vi "Process.vi"(8 "error in":errorcluster, 11 "UI_Generator_Config":refnum<class "UI_Generator_Config.lvclass">) -> (0 "error out":errorcluster, 3 "UI_Generator_Config out":refnum<class "UI_Generator_Config.lvclass">)   [LabVIEW 2016, in "UI_Generator_Config.lvclass"]
doc: "---------------------------------------------------------------\nJKI State Machine Objects™\nhttp://jki.net/state-machine-objects/\nCopyright (C) 2005-2015, JKI <info@jki.net>\nALL RIGHTS RESERVED"
uses:
  UI_Generator_Config.lvclass
  C:/Program Files (x86)/National Instruments/LabVIEW 2016/vi.lib/JKI/JKI SMO/SMO/SMO.lvclass
  Typedefs/AO-cluster.ctl
  Typedefs/AO_Amp-array.ctl
  Typedefs/AO_DC-array.ctl
  Typedefs/AO_f-array.ctl
  Typedefs/AO_phi-array.ctl
  Typedefs/Function-array.ctl
  Typedefs/Function-enum.ctl
  <vilib>/JKI/JKI SMO/SMO/Typedefs/Parent Call--Enum.ctl
  Generator/Typedefs/PrivateEvents--Generator.configGenerator.ctl
  UI_Generator_Config.lvclass/UI_Generator_Config.ctl
  <vilib>/JKI/JKI SMO/SMO/SMO.lvclass
  Generator/Generator.lvclass
panel:
  in  "Channels: AO":T1={"AO amp (V)"=[0.01, 0.0, 0.0, 0.0, 0.0, 0.0, 0.0, 0.0], "AO DC (V)"=[0.0, 0.0, 0.0, 0.0, 0.0, 0.0, 0.0, 0.0], "AO f (Hz)"=[13.1, 13.0, 13.0, 13.0, 13.0, 13.0, 13.0, 13.0], "AO phi (deg)"=[0.0, 0.0, 0.0, 0.0, 0.0, 0.0, 0.0, 0.0], "function"=[enum."Sine Wave", enum."Sine Wave", enum."Sine Wave", enum."Sine Wave", enum."Sine Wave", enum."Sine Wave", enum."Sine Wave", enum."Sine Wave"]} {"AO f (Hz)" min=0.001 max=10000.0; "AO DC (V)" format="%#_6p"; "AO amp (V)" format="%#_6p"}
  in  "Close Window":bool
  # "For instructions on how to use the JKI State Machine Objects, examples and video tutorials, visit:\nhttp://jki.net/state-machine-objects/\n\nJKI State Machine Objects™\nhttp://jki.net/state-machine-objects/\nCopyright (C) 2005-2015, JKI <info@jki.net>\nALL RIGHTS RESERVED"
  # "I think this UI should update Generator live"
  # "configGenerator"
  # "This VI should initialize by asking Generator\nwhat the current settings are...and populating\nthis controls."
  # "0"
  # "1"
  # "2"
  # "3"
  # "4"
  # "5"
  # "6"
  # "7"
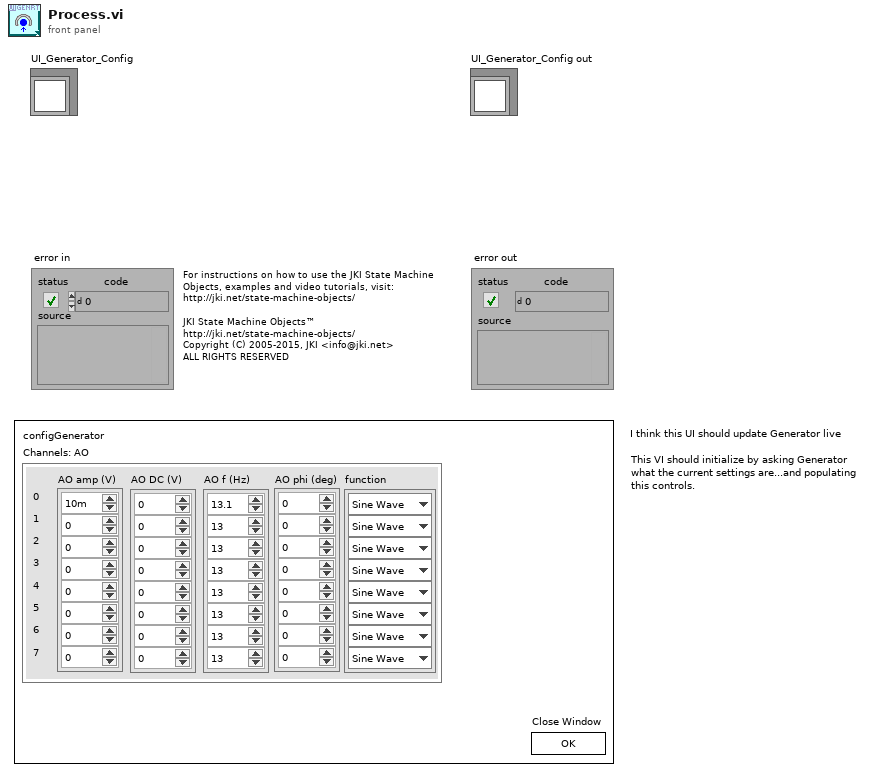
[diagram p1: front panel]
types:
  T1 = typedef "UI_Generator_Config.lvclass/AO-cluster.ctl" = cluster{"AO amp (V)":T2, "AO DC (V)":T3, "AO f (Hz)":T4, "AO phi (deg)":T5, "function":T6}
  T2 = typedef "UI_Generator_Config.lvclass/AO_Amp-array.ctl" = dbl[]
  T3 = typedef "UI_Generator_Config.lvclass/AO_DC-array.ctl" = dbl[]
  T4 = typedef "UI_Generator_Config.lvclass/AO_f-array.ctl" = dbl[]
  T5 = typedef "UI_Generator_Config.lvclass/AO_phi-array.ctl" = dbl[]
  T6 = typedef "UI_Generator_Config.lvclass/Function-array.ctl" = T7[]
  T7 = typedef "UI_Generator_Config.lvclass/Function-enum.ctl" = enum16{"Sine Wave", "Triangle Wave", "Square Wave", "Sawtooth Wave"}
  T8 = cluster{"A (V)":dbl, "DC (V)":dbl, "f (Hz)":dbl, "phi (deg)":dbl, "signal type":enum16{"Sine Wave", "Triangle Wave", "Square Wave", "Sawtooth Wave"}}
  T9 = typedef "SMO.lvclass/Parent Call--Enum.ctl" = enum16{"Allows parent to run", "Does not request parent to run"}
  T10 = enum32{"invalid app kind", "Development System", "Run Time System", "Student Edition", "Embedded LabVIEW", "Evaluation", "Custom"}
  T11 = enum32{"Invalid", "Standard", "Closed", "Hidden", "Minimized", "Maximized"}
  T12 = enum32{"Bad", "Idle", "Run top level", "Running"}
  T13 = typedef "Generator.lvclass/PrivateEvents--Generator.configGenerator.ctl" = cluster{"A (V)":dbl, "DC (V)":dbl, "f (Hz)":dbl, "phi (deg)":dbl, "signal type":enum16{"Sine Wave", "Triangle Wave", "Square Wave", "Sawtooth Wave"}}[]
  T14 = cluster{"Core":cluster{"Current VI Reference":refnum<vi>, "Close Panel on Exit?":bool, "error":errorcluster}, "Self Reference":refnum<class "UI_Generator_Config.lvclass">, "Your string data":string, "configGenerator":T13}
  T15 = cluster{"Current VI Reference":refnum<vi>, "Close Panel on Exit?":bool, "error":errorcluster}
  T16 = typedef "SMO.lvclass/Protected Events.ctl" = cluster{"StopProcesses":refnum<user-event>, "AbortProcesses":refnum<user-event>, "Config Changed":refnum<user-event>, "Dependency":refnum<user-event>}
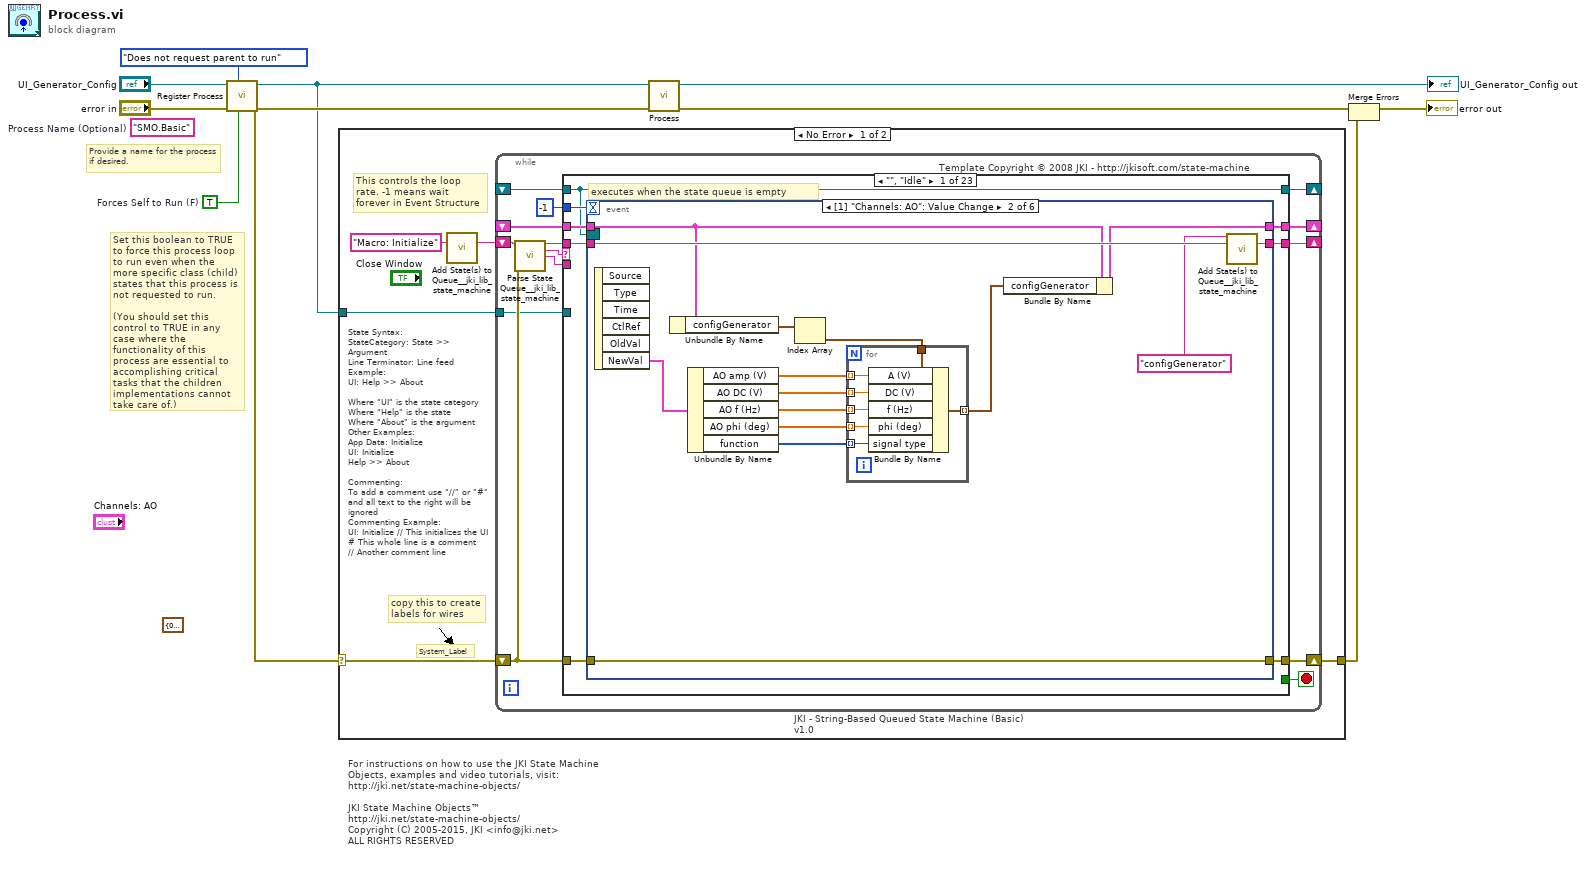
[diagram p0: block diagram]
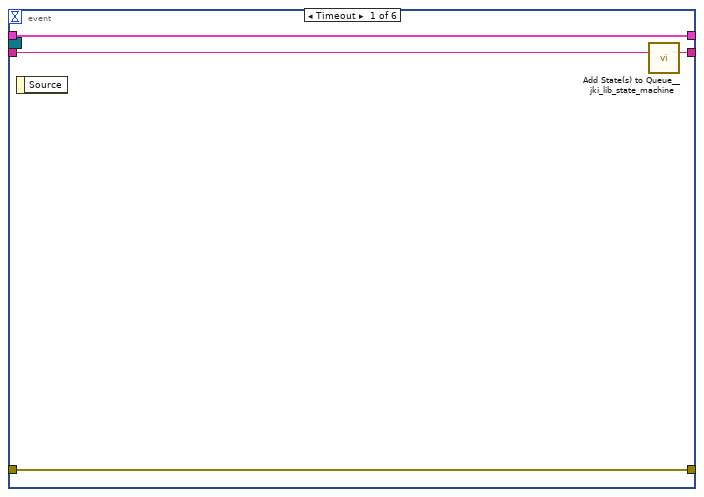
[diagram p2: hidden frame]
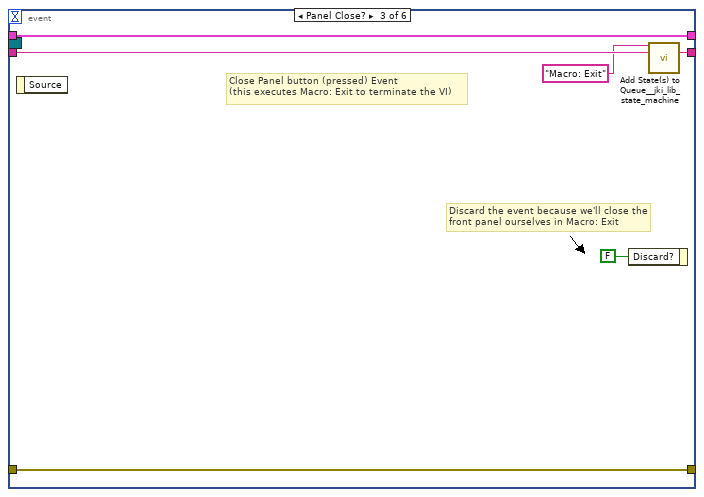
[diagram p3: hidden frame]
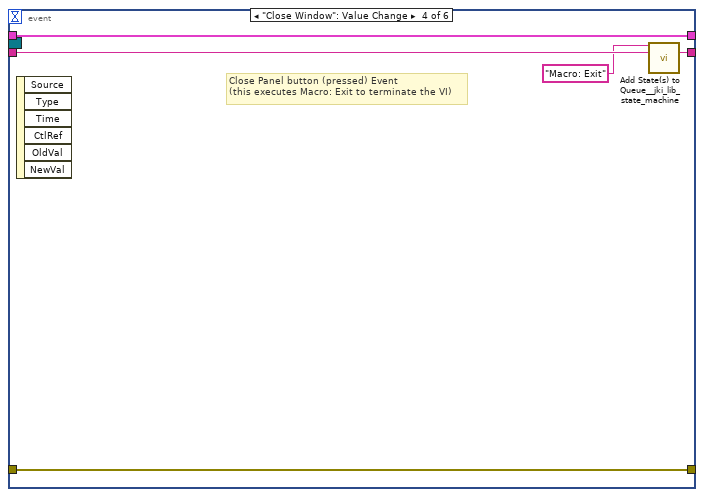
[diagram p4: hidden frame]
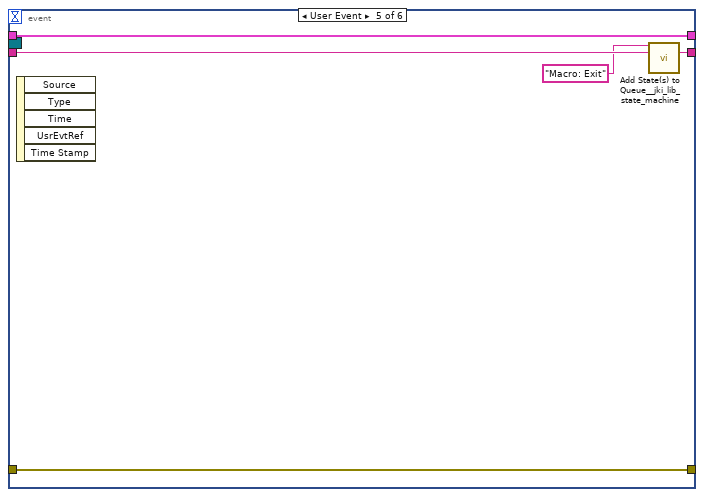
[diagram p5: hidden frame]
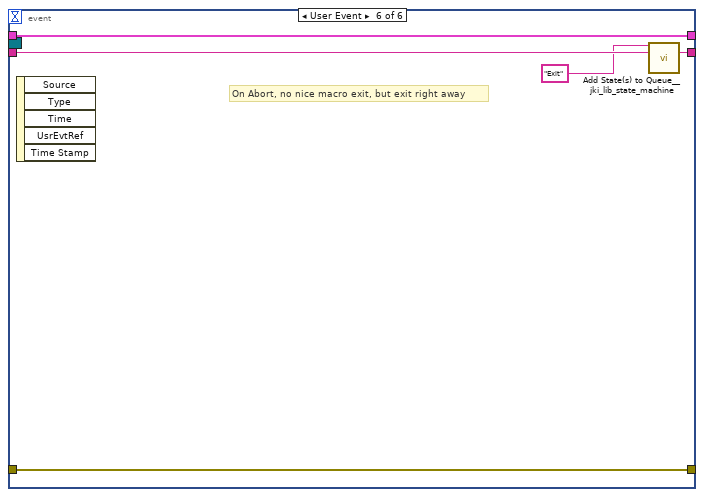
[diagram p6: hidden frame]
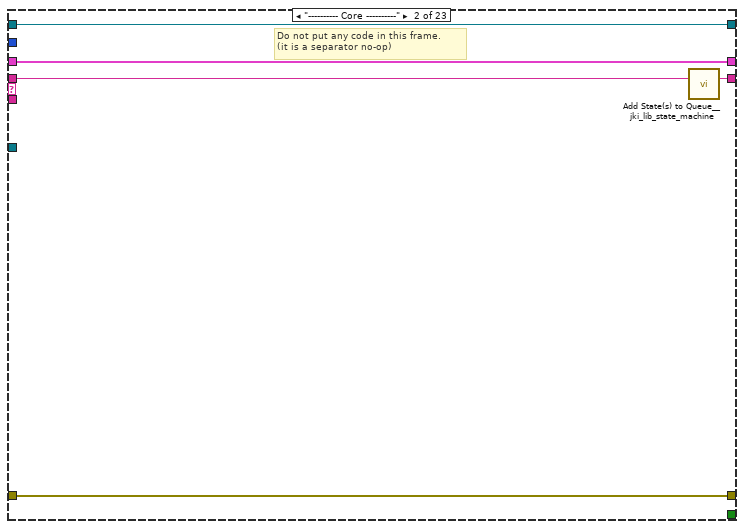
[diagram p7: hidden frame]
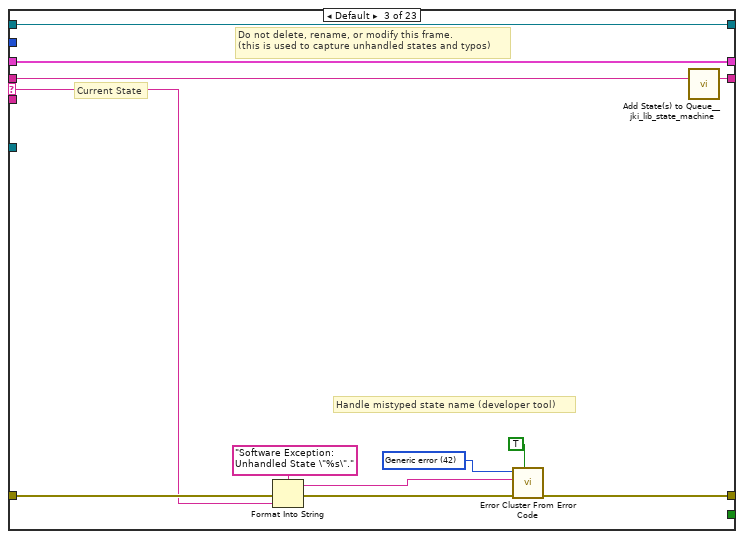
[diagram p8: hidden frame]
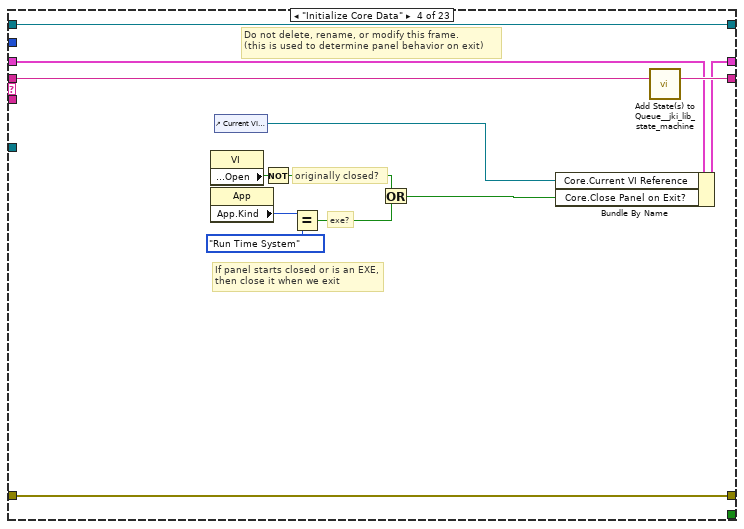
[diagram p9: hidden frame]
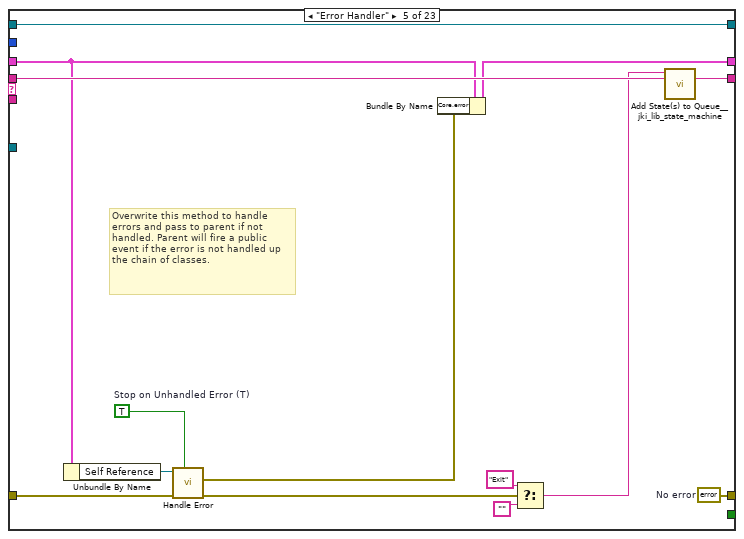
[diagram p10: hidden frame]
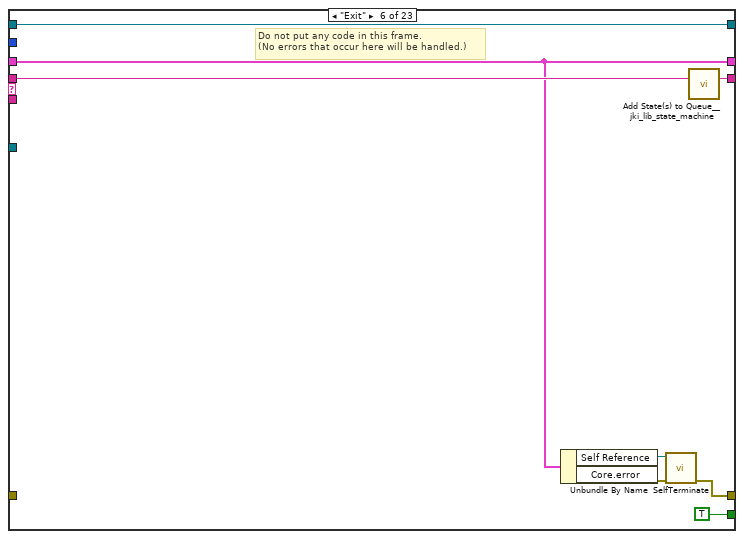
[diagram p11: hidden frame]
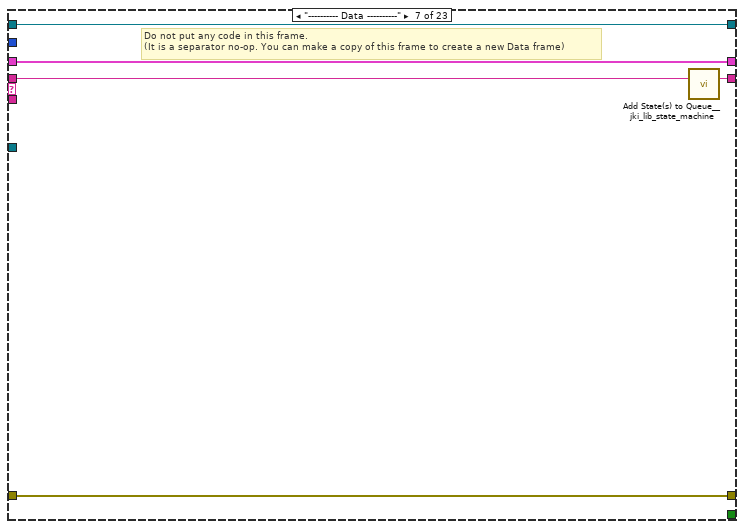
[diagram p12: hidden frame]
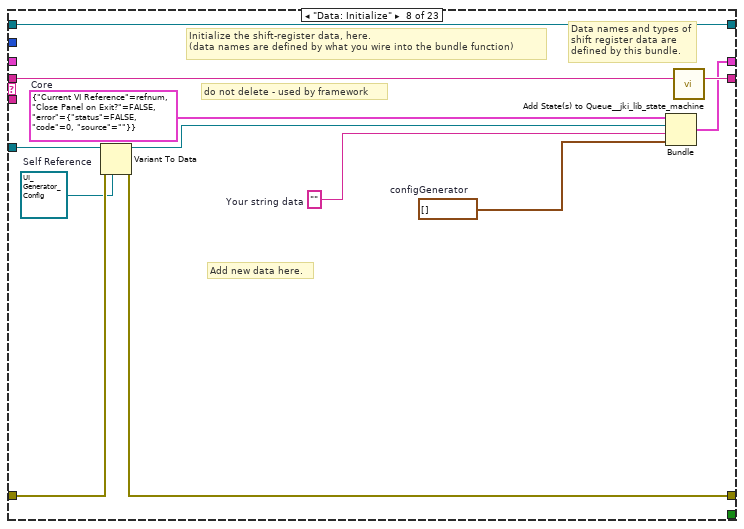
[diagram p13: hidden frame]
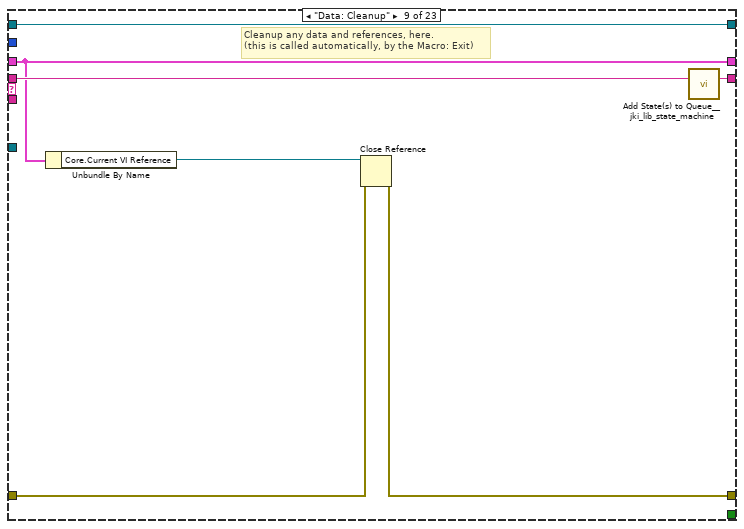
[diagram p14: hidden frame]
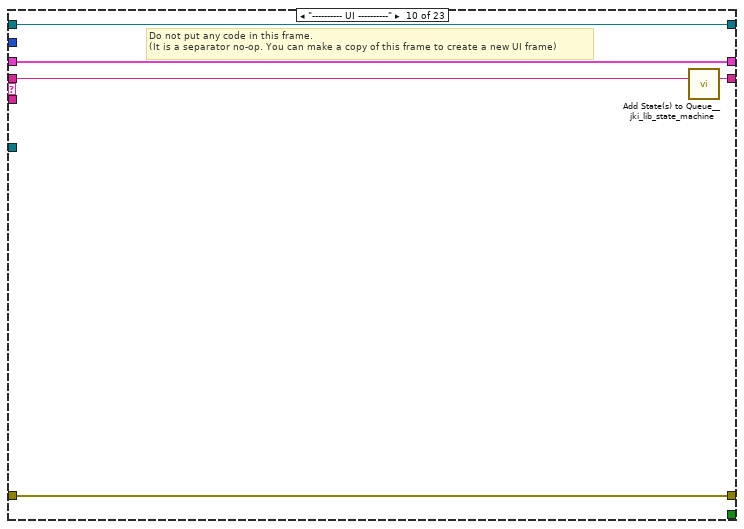
[diagram p15: hidden frame]
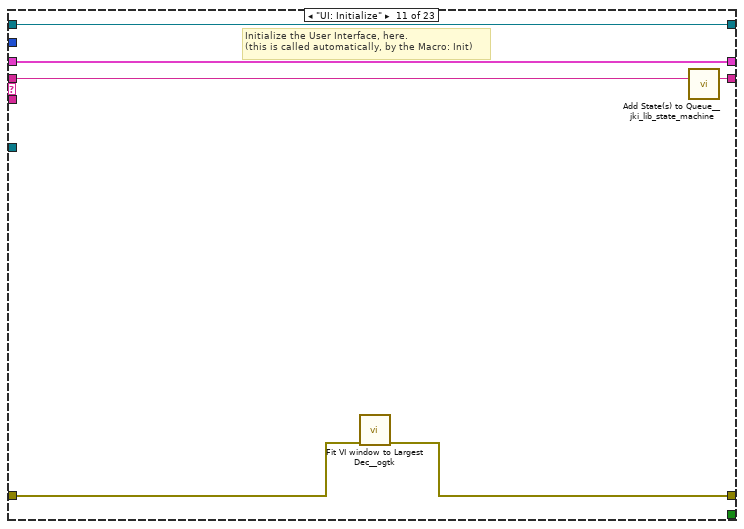
[diagram p16: hidden frame]
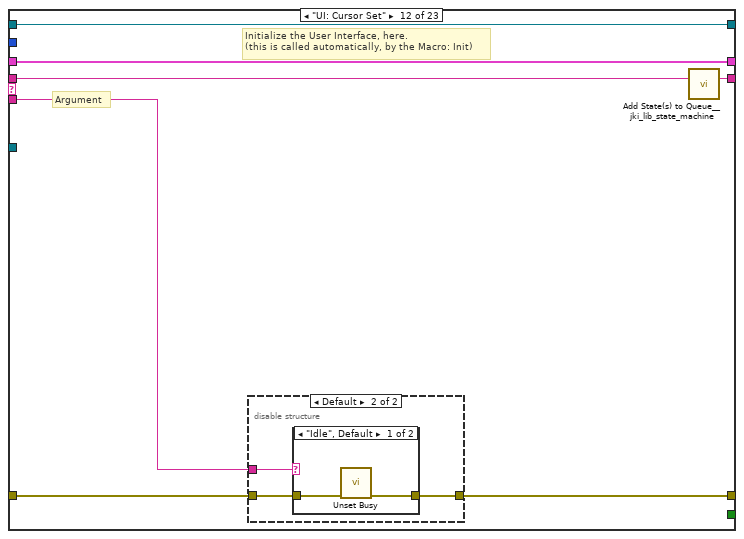
[diagram p17: hidden frame]
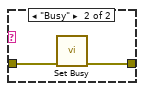
[diagram p19: hidden frame]
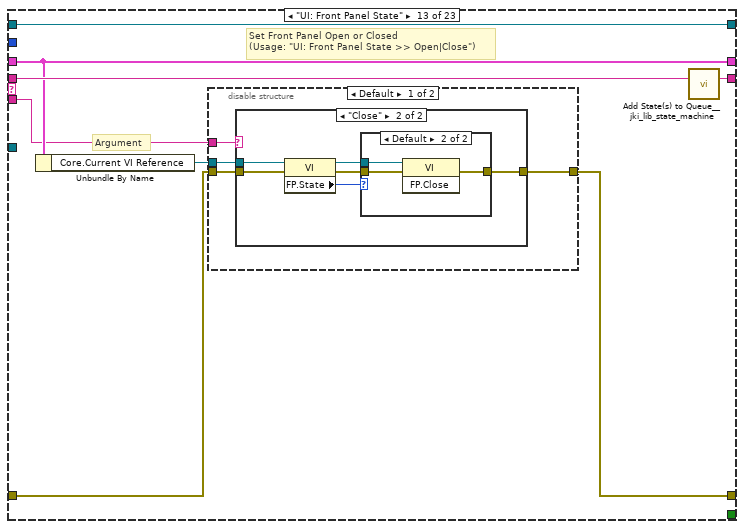
[diagram p20: hidden frame]
diagram:
  (unwired) T8 {"A (V)"=0.0, "DC (V)"=0.0, "f (Hz)"=0.0, "phi (deg)"=0.0, "signal type"=enum."Sine Wave"} ("AO")
  w1 = TRUE  # Forces Self to Run (F)
  (unwired) "SMO.Basic"  # Process Name (Optional)
  # "Provide a name for the process\nif desired."
  # "Set this boolean to TRUE to force this process loop to run even when the more specific class (child) states that this process is not requested to run.\n\n(You should set this control to TRUE in any case where the functionality of this process are essential to accomplishing critical tasks that the children implementations cannot take care of.)"
  # "For instructions on how to use the JKI State Machine Objects, examples and video tutorials, visit:\nhttp://jki.net/state-machine-objects/\n\nJKI State Machine Objects™\nhttp://jki.net/state-machine-objects/\nCopyright (C) 2005-2015, JKI <info@jki.net>\nALL RIGHTS RESERVED"
  n1 = call <vilib>:"Register Process.vi"("Forces Self to Run (F)"=w1, "Parent Call"=Parent_Call--Enum."Does not request parent to run", "error in (no error)"="error in", "SMO"="UI_Generator_Config") -> ("error out"=w7:errorcluster, "SMO out"=w6:refnum<class "UI_Generator_Config.lvclass">)  [unwired: 6 in]
  n2 = case shown="No Error" w7 {
    selector: w7 -> [w12 w304]
    tunnel: w6 -> [w13 _]
    tunnel: [w11 w304] -> w3
    frame No Error {
      # "State Syntax:\nStateCategory: State >> Argument\nLine Terminator: Line feed\nExample:\nUI: Help >> About\n\nWhere \"UI\" is the state category\nWhere \"Help\" is the state\nWhere \"About\" is the argument\nOther Examples:\nApp Data: Initialize\nUI: Initialize\nHelp >> About\n\nCommenting:\nTo add a comment use \"//\" or \"#\" and all text to the right will be ignored\nCommenting Example:\nUI: Initialize // This initializes the UI\n# This whole line is a comment\n// Another comment line"
      # "copy this to create labels for wires"
      # "This controls the loop rate. -1 means wait forever in Event Structure"
      # "System_Label"
      n3 = call <vilib>:"Add State(s) to Queue__jki_lib_state_machine.vi"("State(s) in (\"\")"="Macro: Initialize") -> ("States Out"=w15:string)  [unwired: 14 in]
      n4 = while "JKI - String-Based Queued State Machine (Basic) v1.0" {
        shift-right: [w22] -> _
        shift-left: _ -> [w21]
        shift-right: [w25] -> w11
        shift-left: w12 -> [w19]
        shift-right: [w24] -> _
        shift-left: w15 -> [w26]
        tunnel: w13 -> [w18]
        shift-right: [w17] -> _
        shift-left: _ -> [w16]
        stop <- w23 stop-if-true
        # "Template Copyright © 2008 JKI - http://jkisoft.com/state-machine"
        n5 = call <vilib>:"Parse State Queue__jki_lib_state_machine.vi"("State Queue"=w26, "Error In (no error)"=w19) -> ("Remaining States"=w28:string, "Current State"=w29:string, "Arguments"=w27:string)  [unwired: 11 in]
        n6 = case shown="\"\", \"Idle\"" w29 {
          selector: w29 -> [_ _ w91 _ _ _ _ _ _ _ _ _ _ _ _ _ _ _ _ _ _ _ _]
          tunnel: w28 -> [w37 w89 w95 w114 w128 w136 w141 w153 w160 w165 w171 w178 w194 w226 w240 w254 w259 w270 w275 w285 w291 w296 w303]
          tunnel: w27 -> [_ _ _ _ _ _ _ _ _ _ _ w172 w188 _ _ _ _ _ _ _ _ _ _]
          tunnel: w21 -> [w35 w86 w93 w105 w122 w129 w138 _ w155 w162 w169 w176 w190 w223 w236 w245 w256 w267 w272 w283 w289 w294 w299]
          tunnel: [w34 w87 w97 w111 w123 w130 w139 w148 w156 w163 w166 w173 w191 w224 w238 w252 w257 w261 w273 w278 w287 w292 w300] -> w25
          tunnel: w19 -> [w33 w87 w96 w111 w124 _ w139 w149 w157 w163 w167 w174 w192 w224 w238 w252 w257 w262 w273 w279 w287 w292 w300]
          tunnel: [w36 w88 w94 w113 w127 w135 w140 w152 w159 w164 w170 w177 w193 w225 w239 w253 w258 w269 w274 w284 w290 w295 w302] -> w24
          tunnel: [_ _ _ _ _ TRUE _ _ _ _ _ _ _ _ _ _ _ _ _ _ _ _ _] -> w23
          tunnel: [w32 w86 w93 w112 w121 w129 w138 w151 w155 w162 w169 w176 w190 w223 w236 w245 w256 w267 w272 w283 w289 w294 w299] -> w22
          tunnel: -1 ("Timeout") -> [w31 _ _ _ _ _ _ _ _ _ _ _ _ _ _ _ _ _ _ _ _ _ _]
          tunnel: w18 -> [_ _ _ _ _ _ _ w146 _ _ _ _ _ _ _ _ _ _ _ _ _ _ _]
          tunnel: [w30 w85 w90 w102 w126 w133 w137 w145 w154 w161 w168 w175 w187 w222 w237 w246 w255 w268 w271 w282 w288 w293 w301] -> w17
          tunnel: w16 -> [w30 w85 w90 w102 w126 w133 w137 w145 w154 w161 w168 w175 w187 w222 w237 w246 w255 w268 w271 _ w288 w293 w301]
          frame "", "Idle" {
            # "executes when the state queue is empty"
            n7 = event shown="[1] \"Channels: AO\": Value Change" {
              selector: w30 -> [_ _ _ _ _ _]
              dyn-events: _ -> [_ _ _ _ _ _]
              timeout: w31 -> [_ _ _ _ _ _]
              tunnel: w37 -> [w41 w56 w69 w74 w79 w84]
              tunnel: [w40 w55 w68 w73 w78 w83] -> w36
              tunnel: w35 -> [w39 w51 w66 w71 w76 w81]
              tunnel: [w38 w54 w67 w72 w77 w82] -> w34
              tunnel: w33 -> [w38 w54 w67 w72 w77 w82]
              tunnel: [w39 w53 w66 w71 w76 w81] -> w32
              event Timeout {
                n8 = event-data() -> ()  [unwired: 1 in, 1 out]
                n9 = call <vilib>:"Add State(s) to Queue__jki_lib_state_machine.vi"("State(s) in (\"\")"=w41) -> ("States Out"=w40:string)  [unwired: 14 in]
              }
              event Value Change {
                n10 = event-data() -> ("NewVal"=w52:T1)  [unwired: 1 in, 5 out]
                n11 = Unbundle By Name(w51) -> ("configGenerator"=w50:T13)
                n12 = Unbundle By Name(w52) -> ("AO amp (V)"=w47:T2, "AO DC (V)"=w46:T3, "AO f (Hz)"=w45:T4, "AO phi (deg)"=w44:T5, "function"=w43:T6)
                n13 = Index Array(array=w50) -> (element=w48:T8)  [unwired: 1 in]
                n14 = for {
                  tunnel: w48 -> [w63]
                  tunnel: w47 -> [w62] mode=indexing
                  tunnel: w46 -> [w61] mode=indexing
                  tunnel: w45 -> [w60] mode=indexing
                  tunnel: w44 -> [w59] mode=indexing
                  tunnel: w43 -> [w58] mode=indexing
                  tunnel: [w57] -> w42 mode=indexing
                  n15 = Bundle By Name(cluster=w63, "A (V)"=w62, "DC (V)"=w61, "f (Hz)"=w60, "phi (deg)"=w59, "signal type"=w58) -> (w57:T8)
                }
                n16 = Bundle By Name(cluster=w51, "configGenerator"=w42) -> (w53:T14)
                n17 = call <vilib>:"Add State(s) to Queue__jki_lib_state_machine.vi"("State(s) in Front (\"\")"="configGenerator" ("State(s) in Front (\"\")"), "State(s) in (\"\")"=w56) -> ("States Out"=w55:string)  [unwired: 13 in]
              }
              event Panel Close? {
                # "Discard the event because we'll close the front panel ourselves in Macro: Exit"
                # "Close Panel button (pressed) Event\n(this executes Macro: Exit to terminate the VI)"
                n18 = event-data() -> ()  [unwired: 1 in, 1 out]
                n19 = event-data("Discard?"=FALSE) -> ()  [unwired: 1 in, 1 out]
                n20 = call <vilib>:"Add State(s) to Queue__jki_lib_state_machine.vi"("State(s) in Front (\"\")"="Macro: Exit", "State(s) in (\"\")"=w69) -> ("States Out"=w68:string)  [unwired: 13 in]
              }
              event "Close Window": Value Change {
                # "Close Panel button (pressed) Event\n(this executes Macro: Exit to terminate the VI)"
                n21 = event-data() -> ()  [unwired: 1 in, 6 out]
                n22 = call <vilib>:"Add State(s) to Queue__jki_lib_state_machine.vi"("State(s) in Front (\"\")"="Macro: Exit", "State(s) in (\"\")"=w74) -> ("States Out"=w73:string)  [unwired: 13 in]
              }
              event User Event {
                n23 = event-data() -> ()  [unwired: 1 in, 5 out]
                n24 = call <vilib>:"Add State(s) to Queue__jki_lib_state_machine.vi"("State(s) in Front (\"\")"="Macro: Exit", "State(s) in (\"\")"=w79) -> ("States Out"=w78:string)  [unwired: 13 in]
              }
              event User Event {
                # "On Abort, no nice macro exit, but exit right away"
                n25 = event-data() -> ()  [unwired: 1 in, 5 out]
                n26 = call <vilib>:"Add State(s) to Queue__jki_lib_state_machine.vi"("State(s) in Front (\"\")"="Exit", "State(s) in (\"\")"=w84) -> ("States Out"=w83:string)  [unwired: 13 in]
              }
            }
          }
          frame "---------- Core ----------" {
            # "Do not put any code in this frame.\n(it is a separator no-op)"
            n27 = call <vilib>:"Add State(s) to Queue__jki_lib_state_machine.vi"("State(s) in (\"\")"=w89) -> ("States Out"=w88:string)  [unwired: 14 in]
          }
          frame Default {
            w100 = 42 items=["No error", "Argument error", "Memory is full", "Out of zone", "End of file", "File already open", "Generic file I/O error", "File not found", "File permission error", "Disk is full", "Duplicate path", "Too many files open", "System feature not enabled", "Resource file not found", "Cannot add resource", "Resource not found", "Image not found", "Image memory error", "Pen does not exist", "Config type invalid", "Config token not found", "Config parse error", "Config memory error", "Bad external code format", "Bad external code offset", "External code not present", "Null window", "Destroy window error", "Null menu", "Print aborted", "Bad print record", "Print driver error", "Windows error during printing", "Memory error during printing", "Print dialog error", "Generic print error", "Invalid device refnum", "Device not found", "Device parameter error", "Device unit error", "Cannot open device", "Device call aborted", "Generic error", "Cancelled by user", "Object ID too low", "Object ID too high", "Object not in heap", "Unknown heap", "Unknown object (invalid DefProc)", "Unknown object (DefProc not in table)", "Message out of range", "Invalid (null) method", "Unknown message", "Manager call not supported", "Bad address", "Network operation in progress", "Network operation timed out", "Connection is busy", "Network attribute not supported", "Network error", "Address in use", "System out of memory", "Connection aborted", "Connection refused", "Not connected", "Already connected", "Connection closed", "Initialization error (interapplication manager)", "Bad occurrence", "Wait on unbound occurrence handler", "Occurrence queue overflow", "Datalog type conflict", "Unused", "Unrecognized type (interapplication manager)", "Memory corrupt", "Failed to make temporary DLL", "Old CIN version", "Drag socket not found", "Failed to load drop-object", "Failed to register OLE object", "Failed to release OLE object", "Format specifier type mismatch", "Unknown format specifier", "Too few format specifiers", "Too many format specifiers", "Scan failed", "Newer CIN version", "Error converting to variant", "Runtime menu error", "Password tampered", "Variant attribute not found", "Incompatible variant data type", "Event data is not available", "Event Store is not present", "Occurrence is not found", "Event Queue is not created", "Event info is not available", "Refnum passed is NULL", "Error retrieving Class GUID", "Error retrieving CoClass GUID", "Error retrieving TypeLib GUID.", "Bad built application magic bytes.", "Specific driver is different from the specific driver associated with the Logical Name.", "There is no session opened to the class driver.", "Max Error", "MAX - Error with config objects", "MAX - Error loading configuration", "MAX - Group not supported"]
            # "Current State"
            # "Do not delete, rename, or modify this frame.\n(this is used to capture unhandled states and typos)"
            # "Handle mistyped state name (developer tool)"
            n28 = Format Into String(format string="Software Exception: Unhandled State \"%s\"." ("message"), error in=w96, w91) -> (resulting string=w99:string, error out=w98:errorcluster)  [unwired: 1 in]
            n29 = call <vilib>:"Error Cluster From Error Code.vi"("show call chain? (False)"=TRUE, "error in (no error)"=w98, "error message (\"\")"=w99, "error code (0)"=w100) -> ("error out"=w97:errorcluster)  [unwired: 5 in]
            n30 = call <vilib>:"Add State(s) to Queue__jki_lib_state_machine.vi"("State(s) in (\"\")"=w95) -> ("States Out"=w94:string)  [unwired: 14 in]
          }
          frame "Initialize Core Data" {
            # "Do not delete, rename, or modify this frame.\n(this is used to determine panel behavior on exit)"
            # "originally closed?"
            # "exe?"
            # "If panel starts closed or is an EXE, then close it when we exit"
            n31 = property class="VI"() -> ("Front Panel.Open"=w110:bool)  [unwired: 2 in, 2 out]
            n32 = property class="App"() -> ("App.Kind"=w109:T10)  [unwired: 2 in, 2 out]
            n33 = control-ref of="Current VI Reference"() -> (w103:refnum<vi>)
            n34 = Not(x=w110) -> (.not. x?=w107:bool)
            n35 = Equal?(x=w109, y=T10."Run Time System" ("Application:Kind")) -> (x = y?=w106:bool)
            n36 = Or(x=w107, y=w106) -> (x .or. y?=w104:bool)
            n37 = Bundle By Name(cluster=w105, "Core.Current VI Reference"=w103, "Core.Close Panel on Exit?"=w104) -> (w112:T14)
            n38 = call <vilib>:"Add State(s) to Queue__jki_lib_state_machine.vi"("State(s) in (\"\")"=w114) -> ("States Out"=w113:string)  [unwired: 14 in]
          }
          frame "Error Handler" {
            w115 = TRUE  # Stop on Unhandled Error (T)
            w123 = errorcluster {"status"=FALSE, "code"=0, "source"=""}  # No error
            # "Overwrite this method to handle errors and pass to parent if not handled. Parent will fire a public event if the error is not handled up the chain of classes."
            n39 = Unbundle By Name(w122) -> ("Self Reference"=w125:refnum<class "UI_Generator_Config.lvclass">)
            n40 = call-dynamic "Handle Error.vi"("Stop on Unhandled Error (T)"=w115, "error in"=w124, "SMO"=w125) -> ("handling error"=w116:errorcluster, "Unhandled error"=w119:errorcluster)  [unwired: 6 in, 1 out]
            n41 = Bundle By Name(cluster=w122, "Core.error"=w119) -> (w121:T14)
            n42 = Select(t="Exit", s=w116, f="") -> (s? t:f=w120:string)
            n43 = call <vilib>:"Add State(s) to Queue__jki_lib_state_machine.vi"("State(s) in Front (\"\")"=w120, "State(s) in (\"\")"=w128) -> ("States Out"=w127:string)  [unwired: 13 in]
          }
          frame "Exit" {
            # "Do not put any code in this frame.\n(No errors that occur here will be handled.)"
            n44 = Unbundle By Name(w129) -> ("Self Reference"=w131:refnum<class "UI_Generator_Config.lvclass">, "Core.error"=w132:errorcluster)
            n45 = call <vilib>:"SelfTerminate.vi"("error in (no error)"=w132, "SMO in"=w131) -> ("error out"=w130:errorcluster)  [unwired: 8 in, 1 out]
            n46 = call <vilib>:"Add State(s) to Queue__jki_lib_state_machine.vi"("State(s) in (\"\")"=w136) -> ("States Out"=w135:string)  [unwired: 14 in]
          }
          frame "---------- Data ----------" {
            # "Do not put any code in this frame.\n(It is a separator no-op. You can make a copy of this frame to create a new Data frame)"
            n47 = call <vilib>:"Add State(s) to Queue__jki_lib_state_machine.vi"("State(s) in (\"\")"=w141) -> ("States Out"=w140:string)  [unwired: 14 in]
          }
          frame "Data: Initialize" {
            w142 = T13 []  # configGenerator
            w144 = T15 {"Current VI Reference"=refnum, "Close Panel on Exit?"=FALSE, "error"={"status"=FALSE, "code"=0, "source"=""}}  # Core
            w147 = refnum<class "UI_Generator_Config.lvclass"> refnum  # Self Reference
            w150 = ""  # Your string data
            # "do not delete - used by framework"
            # "Add new data here."
            # "Data names and types of shift register data are defined by this bundle."
            # "Initialize the shift-register data, here.\n(data names are defined by what you wire into the bundle function)"
            n48 = Variant To Data(error in=w149, type=w147, Variant=w146) -> (data=w143:refnum<class "UI_Generator_Config.lvclass">, error out=w148:errorcluster)
            n49 = Bundle("Core"=w144, "Self Reference"=w143, "Your string data"=w150, "configGenerator"=w142) -> (w151:T14)  [unwired: 1 in]
            n50 = call <vilib>:"Add State(s) to Queue__jki_lib_state_machine.vi"("State(s) in (\"\")"=w153) -> ("States Out"=w152:string)  [unwired: 14 in]
          }
          frame "Data: Cleanup" {
            # "Cleanup any data and references, here.\n(this is called automatically, by the Macro: Exit)"
            n51 = Unbundle By Name(w155) -> ("Core.Current VI Reference"=w158:refnum<vi>)
            n52 = Close Reference(reference=w158, error in (no error)=w157) -> (error out=w156:errorcluster)
            n53 = call <vilib>:"Add State(s) to Queue__jki_lib_state_machine.vi"("State(s) in (\"\")"=w160) -> ("States Out"=w159:string)  [unwired: 14 in]
          }
          frame "---------- UI ----------" {
            # "Do not put any code in this frame.\n(It is a separator no-op. You can make a copy of this frame to create a new UI frame)"
            n54 = call <vilib>:"Add State(s) to Queue__jki_lib_state_machine.vi"("State(s) in (\"\")"=w165) -> ("States Out"=w164:string)  [unwired: 14 in]
          }
          frame "UI: Initialize" {
            # "Initialize the User Interface, here.\n(this is called automatically, by the Macro: Init)"
            n55 = call <userlib>:"Fit VI window to Largest Dec__ogtk.vi"("error in (no error)"=w167) -> ("error out"=w166:errorcluster)  [unwired: 5 in, 1 out]
            n56 = call <vilib>:"Add State(s) to Queue__jki_lib_state_machine.vi"("State(s) in (\"\")"=w171) -> ("States Out"=w170:string)  [unwired: 14 in]
          }
          frame "UI: Cursor Set" {
            # "Argument"
            # "Initialize the User Interface, here.\n(this is called automatically, by the Macro: Init)"
            n57 = disable-structure shown="Default" {
              disable-tunnel: w174 -> [w179 w182]
              disable-tunnel: [w179 w181] -> w173
              disable-tunnel: w172 -> [_ w180]
              frame condition #0 {
              }
              frame condition #1 (active) {
                n58 = case shown="\"Idle\", Default" w180 {
                  tunnel: w182 -> [w184 w186]
                  tunnel: [w183 w185] -> w181
                  frame "Idle", Default {
                    n59 = call <vilib>:"Unset Busy.vi"("error in (no error)"=w184) -> ("error out"=w183:errorcluster)  [unwired: 10 in]
                  }
                  frame "Busy" {
                    n60 = call <vilib>:"Set Busy.vi"("error in (no error)"=w186) -> ("error out"=w185:errorcluster)  [unwired: 9 in, 1 out]
                  }
                }
              }
            }
            n61 = call <vilib>:"Add State(s) to Queue__jki_lib_state_machine.vi"("State(s) in (\"\")"=w178) -> ("States Out"=w177:string)  [unwired: 14 in]
          }
          frame "UI: Front Panel State" {
            # "Argument"
            # "Set Front Panel Open or Closed\n(Usage: \"UI: Front Panel State >> Open|Close\")"
            n62 = Unbundle By Name(w190) -> ("Core.Current VI Reference"=w189:refnum<vi>)
            n63 = disable-structure shown="Default" {
              disable-tunnel: w192 -> [w198 w221]
              disable-tunnel: [w197 w221] -> w191
              disable-tunnel: w189 -> [w196 _]
              disable-tunnel: w188 -> [w195 _]
              frame condition #0 (active) {
                n64 = case shown="\"Close\"" w195 {
                  tunnel: w198 -> [w202 w215]
                  tunnel: [w204 w216] -> w197
                  tunnel: w196 -> [w203 w213]
                  frame "Open", Default {
                    n65 = property class="VI"(reference=w203, error in=w202) -> (reference out=w200:refnum<vi>, error out=w201:errorcluster, "FP.State"=w199:T11)
                    n66 = case shown="\"Closed\"" w199 {
                      tunnel: [w207 w210] -> w204
                      tunnel: w201 -> [w206 w210]
                      tunnel: w200 -> [w205 _]
                      frame "Closed" {
                        n67 = invoke class="VI" method="FP.Open"(reference=w205, error in=w206, "Activate"=TRUE, "State"=T11."Standard") -> (error out=w207:errorcluster)  [unwired: 1 in, 4 out]
                      }
                      frame Default {
                      }
                    }
                  }
                  frame "Close" {
                    n68 = property class="VI"(reference=w213, error in=w215) -> (reference out=w212:refnum<vi>, error out=w214:errorcluster, "FP.State"=w211:T11)
                    n69 = case shown="Default" w211 {
                      tunnel: [w217 w220] -> w216
                      tunnel: w214 -> [w217 w219]
                      tunnel: w212 -> [_ w218]
                      frame "Invalid", "Closed" {
                      }
                      frame Default {
                        n70 = invoke class="VI" method="FP.Close"(reference=w218, error in=w219) -> (error out=w220:errorcluster)  [unwired: 1 in, 2 out]
                      }
                    }
                  }
                }
              }
              frame condition #1 {
              }
            }
            n71 = call <vilib>:"Add State(s) to Queue__jki_lib_state_machine.vi"("State(s) in (\"\")"=w194) -> ("States Out"=w193:string)  [unwired: 14 in]
          }
          frame "---------- Macro ----------" {
            # "Do not put any code in this frame.\n(It is a separator no-op. You can make a copy of this frame to create a new Macro frame)"
            n72 = call <vilib>:"Add State(s) to Queue__jki_lib_state_machine.vi"("State(s) in (\"\")"=w226) -> ("States Out"=w225:string)  [unwired: 14 in]
          }
          frame "Macro: Initialize" {
            w231 = "UI: Initialize\nUI: Front Panel State >> Open"  # UI: Initialize UI: Front Panel State >> Open
            w227 = "Process: Sync"
            # "Initialization Macro\n(This is called once, when the VI starts)"
            n73 = control-ref of="This VI"() -> (w229:refnum<vi>)
            n74 = property class="VI"(reference=w229) -> ("Exec.State"=w228:T12)  [unwired: 1 in, 2 out]
            n75 = Equal?(x=w228, y=T12."Run top level") -> (x = y?=w234:bool)
            n76 = Select(t=w227, s=w234, f="") -> ()  [unwired: 1 out]
            n77 = call <vilib>:"Add State(s) to Queue__jki_lib_state_machine.vi"("State(s) in Front (\"\")"="Data: Initialize\nInitialize Core Data\nEvents: Register", "State(s) in (\"\")"=w227, "State(s) at Back (\"\")"=w231) -> ("States Out"=w230:string)  [unwired: 12 in]
            n78 = call <vilib>:"Add State(s) to Queue__jki_lib_state_machine.vi"("State(s) in Front (\"\")"=w230, "State(s) in (\"\")"=w240) -> ("States Out"=w239:string)  [unwired: 13 in]
          }
          frame "Macro: Exit" {
            # "Exit Macro\n(This is called once, when the VI exits)"
            n79 = Unbundle By Name(w245) -> ("Core.Close Panel on Exit?"=w251:bool)
            n80 = Select(t="UI: Front Panel State >> Close", s=w251, f="") -> (s? t:f=w248:string)
            n81 = call <vilib>:"Add State(s) to Queue__jki_lib_state_machine.vi"("State(s) in Front (\"\")"="Data: Cleanup\nEvents: Unregister", "State(s) in (\"\")"="Process: Sync", "State(s) at Back (\"\")"="Exit") -> ("States Out"=w242:string)  [unwired: 12 in]
            n82 = call <vilib>:"Add State(s) to Queue__jki_lib_state_machine.vi"("State(s) in (\"\")"=w248, "State(s) at Back (\"\")"=w242) -> ("States Out"=w247:string)  [unwired: 13 in]
            n83 = call <vilib>:"Add State(s) to Queue__jki_lib_state_machine.vi"("State(s) in Front (\"\")"=w247, "State(s) in (\"\")"=w254) -> ("States Out"=w253:string)  [unwired: 13 in]
          }
          frame "---------- Process ----------" {
            # "Template Separator\n(You can make a copy of, or modify, this frame)"
            n84 = call <vilib>:"Add State(s) to Queue__jki_lib_state_machine.vi"("State(s) in (\"\")"=w259) -> ("States Out"=w258:string)  [unwired: 14 in]
          }
          frame "Process: Sync" {
            n85 = Unbundle By Name(w267) -> ("Self Reference"=w263:refnum<class "UI_Generator_Config.lvclass">)
            n86 = call <vilib>:"WaitOnProcessSync.vi"("error in (no error)"=w262, "SMO"=w263) -> ("error out"=w261:errorcluster, "Don't run?"=w266:bool)  [unwired: 7 in, 1 out]
            n87 = Select(t="Data: Cleanup\nEvents: Unregister\nExit", s=w266, f="") -> (s? t:f=w260:string)
            n88 = call <vilib>:"Add State(s) to Queue__jki_lib_state_machine.vi"("State(s) in Front (\"\")"=w260, "State(s) in (\"\")"=w270) -> ("States Out"=w269:string)  [unwired: 13 in]
          }
          frame "---------- Events ----------" {
            # "Template Separator\n(You can make a copy of, or modify, this frame)"
            n89 = call <vilib>:"Add State(s) to Queue__jki_lib_state_machine.vi"("State(s) in (\"\")"=w275) -> ("States Out"=w274:string)  [unwired: 14 in]
          }
          frame "Events: Register" {
            # "Expand to add\nmore events"
            n90 = Unbundle By Name(w283) -> ("Self Reference"=w280:refnum<class "UI_Generator_Config.lvclass">)
            n91 = call <vilib>:"GetProtectedEvents.vi"("SMO"=w280) -> ("error out"=w276:errorcluster, "SMO Protected Events"=w281:T16)  [unwired: 8 in, 1 out]
            n92 = register-events(w281) -> (reference out=w282:refnum<event-registration>, error out=w277:errorcluster)  [unwired: 2 in]
            n93 = Merge Errors(w279, w277, w276) -> (w278:errorcluster)
            n94 = call <vilib>:"Add State(s) to Queue__jki_lib_state_machine.vi"("State(s) in (\"\")"=w285) -> ("States Out"=w284:string)  [unwired: 14 in]
          }
          frame "Events: Unregister" {
            n95 = Unregister For Events(event registration refnum=w288, error in=w287) -> (error out=w286:errorcluster)
            n96 = call <vilib>:"Clear Errors.vi"("error in (no error)"=w286) -> ()  [unwired: 5 in, 2 out]
            n97 = call <vilib>:"Add State(s) to Queue__jki_lib_state_machine.vi"("State(s) in (\"\")"=w291) -> ("States Out"=w290:string)  [unwired: 14 in]
          }
          frame "---------- Action ----------" {
            n98 = call <vilib>:"Add State(s) to Queue__jki_lib_state_machine.vi"("State(s) in (\"\")"=w296) -> ("States Out"=w295:string)  [unwired: 14 in]
          }
          frame "configGenerator" {
            n99 = Unbundle By Name(w299) -> ("Self Reference"=w298:refnum<class "UI_Generator_Config.lvclass">)  [unwired: 1 out]
            n100 = Unbundle By Name(w298) -> ("Generator"=w297:refnum<class "Generator.lvclass">)
            n101 = call "Generator.configGenerator.vi"("Generator"=w297) -> ()  [unwired: 9 in, 2 out]
            n102 = call <vilib>:"Add State(s) to Queue__jki_lib_state_machine.vi"("State(s) in (\"\")"=w303) -> ("States Out"=w302:string)  [unwired: 14 in]
          }
        }
      }
    }
    frame Error {
    }
  }
  n103 = call-parent "Process.vi"("error in"=w7, "SMO"=w6) -> ("error out"=w4:errorcluster, "SMO out"=→"UI_Generator_Config out":refnum<class "UI_Generator_Config.lvclass">)  [unwired: 8 in]
  n104 = Merge Errors(w4, w3) -> (→"error out":errorcluster)
